vi "PropertyListAddControls.vi"(7 "Indentation":i32, 8 "error in (no error)":errorcluster, 9 "Path":string, 10 "Controls[]":refnum<vi>[](array[refnum]), 11 "TreeControl in":refnum<vi>) -> (3 "TreeControl out":refnum<vi>)   [LabVIEW 2021, in "VIPropertyPicker.lvlib"]
uses:
  VIPropertyPicker.lvlib
  lib/SetGetControlValue/SetGetControlValue.lvlib
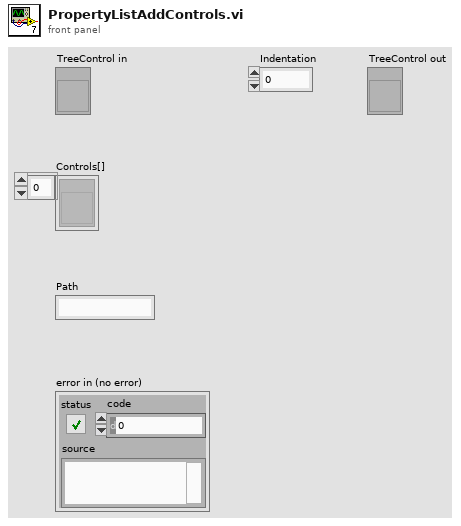
[diagram p1: front panel]
types:
  T1 = enum8{"Enabled", "Disabled", "Disabled and Grayed Out"}
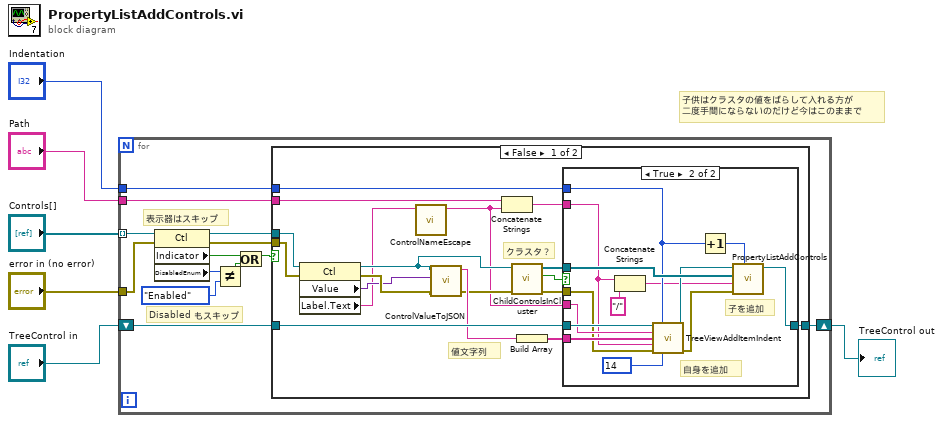
[diagram p0: block diagram]
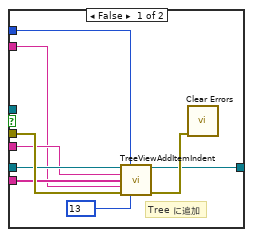
[diagram p2: hidden frame]
diagram:
  # "子供はクラスタの値をばらして入れる方が\n二度手間にならないのだけど今はこのままで"
  n1 = for {
    shift-right: [w17] -> w5
    shift-left: "TreeControl in" -> [w16]
    tunnel: "Controls[]" -> [w15] mode=indexing
    tunnel: "Path" -> [w19]
    tunnel: "Indentation" -> [w18]
    tunnel: "error in (no error)" -> [w13]
    # "Disabled もスキップ"
    # "表示器はスキップ"
    n2 = property class="Ctl"(reference=w15, error in=w13) -> (reference out=w14:refnum<vi>, error out=w12:errorcluster, "Indicator"=w11:bool, "DisabledEnum"=w10:T1)
    n3 = Not Equal?(x=w10, y=T1."Enabled" ("Disabled")) -> (x != y?=w7:bool)
    n4 = Or(x=w11, y=w7) -> (x .or. y?=w8:bool)
    n5 = case shown="False" w8 {
      tunnel: w19 -> [w37 _]
      tunnel: w18 -> [w32 _]
      tunnel: [w31 w61] -> w17
      tunnel: w16 -> [w30 w61]
      tunnel: w14 -> [w28 _]
      tunnel: w12 -> [w27 _]
      frame False {
        # "値文字列"
        # "クラスタ？"
        n6 = property class="Ctl"(reference=w28, error in=w27) -> (reference out=w25:refnum<vi>, error out=w26:errorcluster, "Value"=w22:variant, "Label.Text"=w21:string)
        n7 = call "ControlNameEscape.vi"("label"=w21) -> ("escaped string"=w20:string)  [unwired: 10 in]
        n8 = call "ControlValueToJSON.vi"("error in (no error)"=w26, "Value"=w22, "Control in"=w25) -> ("error out"=w23:errorcluster, "String"=w24:string)  [unwired: 7 in]
        n9 = Concatenate Strings(w37, w20) -> (w34:string)
        n10 = call "ChildControlsInCluster.vi"("error in (no error)"=w23, "Control in"=w25) -> ("error out"=w33:errorcluster, "IsCluster"=w36:bool, "Controls[]"=w35:refnum<vi>[])  [unwired: 7 in]
        n11 = Build Array(w24) -> (w29:string[])
        n12 = case shown="True" w36 {
          tunnel: w35 -> [_ w60]
          tunnel: w34 -> [w40 w50]
          tunnel: w33 -> [w46 w52]
          tunnel: w32 -> [w39 w56]
          tunnel: [w44 w58] -> w31
          tunnel: w30 -> [w43 w57]
          tunnel: w20 -> [w42 w55]
          tunnel: w29 -> [w41 w54]
          frame False {
            # "Tree に追加"
            n13 = call "TreeViewAddItemIndent.vi"("TreeControl in"=w43, "Indentation"=w39, "Left Cell String"=w42, "Child Text"=w41, "Tag"=w40, "error in (no error)"=w46, "Symbol Index"=13) -> ("TreeControl out"=w44:refnum<vi>, "error out"=w45:errorcluster)  [unwired: 6 in, 1 out]
            n14 = call <vilib>:"Clear Errors.vi"("error in (no error)"=w45) -> ()  [unwired: 5 in, 2 out]
          }
          frame True {
            # "子を追加"
            # "自身を追加"
            n15 = Concatenate Strings(w50, "/" ("string")) -> (w49:string)
            n16 = call "TreeViewAddItemIndent.vi"("TreeControl in"=w57, "Indentation"=w56, "Left Cell String"=w55, "Child Text"=w54, "Tag"=w50, "error in (no error)"=w52, "Symbol Index"=14) -> ("TreeControl out"=w53:refnum<vi>, "error out"=w51:errorcluster)  [unwired: 6 in, 1 out]
            n17 = Increment(x=w56) -> (x+1=w59:i32)
            n18 = call "PropertyListAddControls.vi"("Indentation"=w59, "error in (no error)"=w51, "Path"=w49, "Controls[]"=w60, "TreeControl in"=w53) -> ("TreeControl out"=w58:refnum<vi>)  [unwired: 6 in]
          }
        }
      }
      frame True {
      }
    }
  }
  "TreeControl out" <- w5
